vi "Orientation Angle.vi"(8 "Refractive Index (Dense)":dbl, 9 "Refractive Index (Rare)":dbl, 10 "Dichroic Ratio":dbl, 11 "Incident Angle (Degrees)":dbl) -> (3 "Orientation Angle (Degrees)":dbl)   [LabVIEW 2017, in "LD Reading.lvclass"]
uses:
  LD Reading.lvclass
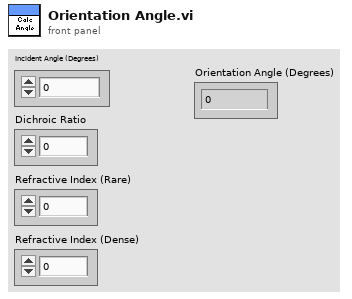
[diagram p1: front panel]
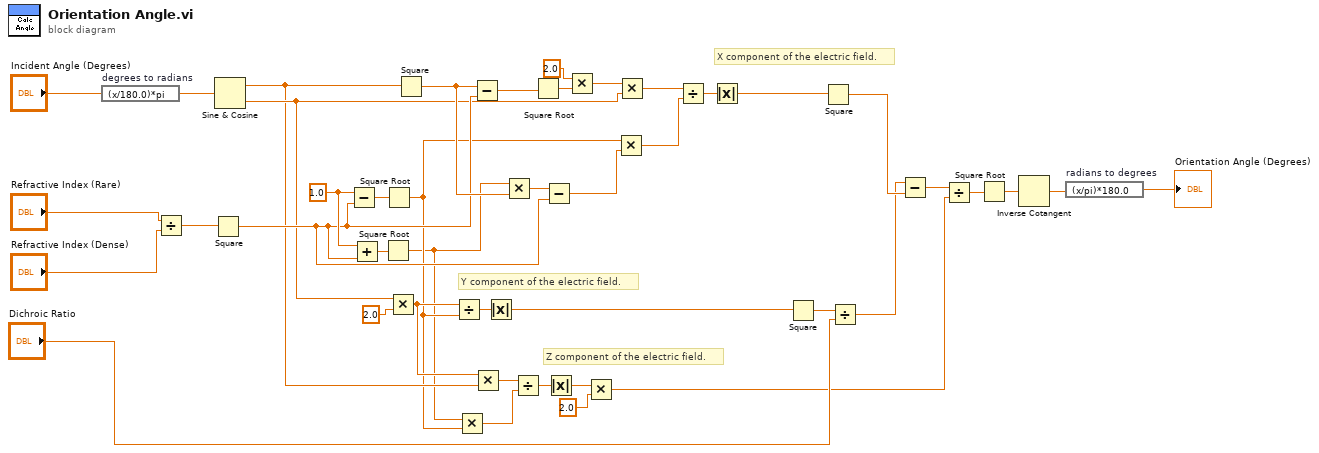
[diagram p0: block diagram]
diagram:
  w32 = 1.0 ("x")
  # "Z component of the electric field."
  # "Y component of the electric field."
  # "X component of the electric field."
  n1 = expression code="(x/180.0)*pi" "degrees to radians"("Incident Angle (Degrees)") -> (w40:dbl)
  n2 = Divide(x="Refractive Index (Rare)", y="Refractive Index (Dense)") -> (x/y=w39:dbl)
  n3 = Square(x=w39) -> (x^2=w28:dbl)
  n4 = Sine & Cosine(0:w40) -> (1:w20:dbl, 2:w24:dbl)
  n5 = Subtract(x=w32, y=w28) -> (x-y=w33:dbl)
  n6 = Add(x=w32, y=w28) -> (x+y=w31:dbl)
  n7 = Square Root(x=w31) -> (sqrt(x)=w17:dbl)
  n8 = Square Root(x=w33) -> (sqrt(x)=w18:dbl)
  n9 = Multiply(x=w24, y=2.0 ("x")) -> (x*y=w21:dbl)
  n10 = Square(x=w20) -> (x^2=w30:dbl)
  n11 = Divide(x=w21, y=w18) -> (x/y=w22:dbl)
  n12 = Multiply(x=w17, y=w18) -> (x*y=w16:dbl)
  n13 = Subtract(x=w30, y=w28) -> (x-y=w38:dbl)
  n14 = Multiply(x=w21, y=w20) -> (x*y=w19:dbl)
  n15 = Absolute Value(x=w22) -> (abs(x)=w14:dbl)
  n16 = Multiply(x=w17, y=w30) -> (x*y=w29:dbl)
  n17 = Divide(x=w19, y=w16) -> (x/y=w15:dbl)
  n18 = Square Root(x=w38) -> (sqrt(x)=w37:dbl)
  n19 = Subtract(x=w29, y=w28) -> (x-y=w27:dbl)
  n20 = Absolute Value(x=w15) -> (abs(x)=w8:dbl)
  n21 = Multiply(x=2.0, y=w37) -> (x*y=w35:dbl)
  n22 = Multiply(x=w8, y=2.0 ("x")) -> (x*y=w5:dbl)
  n23 = Multiply(x=w18, y=w27) -> (x*y=w26:dbl)
  n24 = Multiply(x=w35, y=w24) -> (x*y=w34:dbl)
  n25 = Divide(x=w34, y=w26) -> (x/y=w23:dbl)
  n26 = Absolute Value(x=w23) -> (abs(x)=w11:dbl)
  n27 = Square(x=w14) -> (x^2=w13:dbl)
  n28 = Square(x=w11) -> (x^2=w10:dbl)
  n29 = Divide(x=w13, y="Dichroic Ratio") -> (x/y=w9:dbl)
  n30 = Subtract(x=w9, y=w10) -> (x-y=w6:dbl)
  n31 = Divide(x=w6, y=w5) -> (x/y=w4:dbl)
  n32 = Square Root(x=w4) -> (sqrt(x)=w3:dbl)
  n33 = Inverse Cotangent(1:w3) -> (0:w2:dbl)
  n34 = expression code="(x/pi)*180.0" "radians to degrees"(w2) -> (→"Orientation Angle (Degrees)":dbl)
